vi "Self Configure.vi"(8 "error in":errorcluster, 11 "CrossPoint in":refnum<class "CrossPoint.lvclass">) -> (0 "error out":errorcluster, 3 "CrossPoint out":refnum<class "CrossPoint.lvclass">)   [LabVIEW 2019, in "CrossPoint.lvlib" / "CrossPoint.lvclass"]
doc: "Children of Instruments must override this routine and call the parent method. \nThis routine is implemented to allow each instrument to read its specific configuration keys and implement any default configuration settings.\n\nThis routine already calls Connect and Self Test Routines."
uses:
  Library/CrossPoint.lvclass
  Custom Controls/Configuration Keys.ctl
  Library/CrossPoint.lvclass/CrossPoint.ctl
  builds/Instruments/Instruments.lvlibp/Library/Instruments.lvclass
  builds/Tools/Config.lvlibp/Config.lvclass
  C:/Users/Public/Documents/Development/builds/Tools/Config.lvlibp/Config.lvclass
panel:
  in  "Configuration Keys":T1
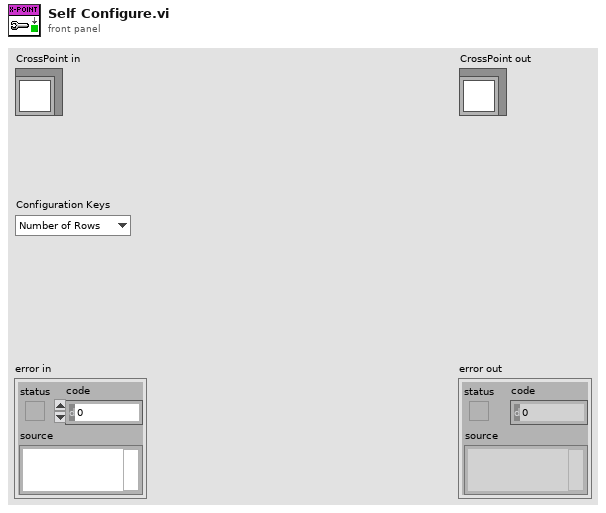
[diagram p1: front panel]
types:
  T1 = typedef "CrossPoint.lvlib/CrossPoint.lvclass/Configuration Keys.ctl" = enum16{"Number of Rows", "Number of Columns"}
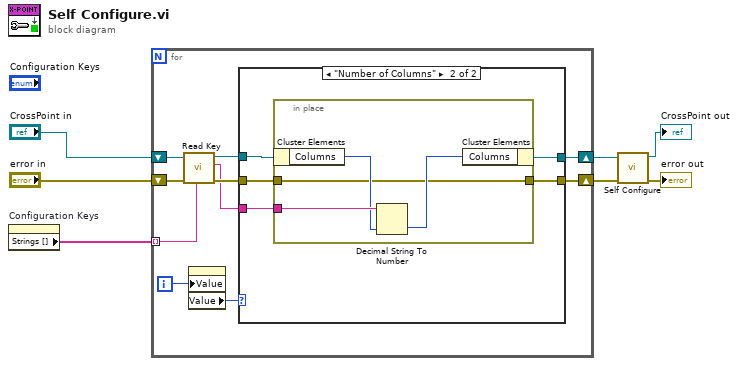
[diagram p0: block diagram]
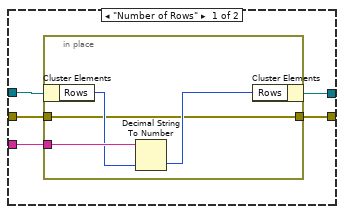
[diagram p2: hidden frame]
diagram:
  n1 = property on="Configuration Keys" class="Enum (strict)"() -> ("Strings []"=w1:string[])  [unwired: 2 in, 2 out]
  n2 = for {
    shift-right: [w10] -> w4
    shift-left: "CrossPoint in" -> [w15]
    shift-right: [w8] -> w2
    shift-left: "error in" -> [w14]
    tunnel: w1 -> [w13] mode=indexing
    i -> [w17]
    n3 = call "Read Key.vi"("Key Name"=w13, "error in"=w14, "Config in"=w15) -> ("error out"=w12:errorcluster, "Key Value"=w9:string, "Config out"=w11:refnum<class "CrossPoint.lvclass">)  [unwired: 6 in]
    n4 = property on="Configuration Keys" class="Enum (strict)"("Value"=w17) -> ("Value"=w16:T1)  [unwired: 2 in, 2 out]
    n5 = case shown="\"Number of Columns\"" w16 {
      tunnel: w12 -> [w20 w29]
      tunnel: w11 -> [w22 w31]
      tunnel: [w21 w30] -> w10
      tunnel: w9 -> [w19 w28]
      tunnel: [w18 w27] -> w8
      frame "Number of Rows" {
        n6 = in-place {
          in-place-border: w20 -> [w23]
          in-place-border: w19 -> [w26]
          in-place-border: [w23] -> w18
          n7 = in-place-cluster #1(w22) -> ("Rows"=w25:u32)
          n8 = Decimal String To Number(string=w26, default (0L)=w25) -> (number=w24:u32)  [unwired: 1 in, 1 out]
          n9 = in-place-cluster #1("Rows"=w24) -> (w21:refnum<class "CrossPoint.lvclass">)
        }
      }
      frame "Number of Columns" {
        n10 = in-place {
          in-place-border: w29 -> [w32]
          in-place-border: w28 -> [w35]
          in-place-border: [w32] -> w27
          n11 = in-place-cluster #2(w31) -> ("Columns"=w34:u32)
          n12 = Decimal String To Number(string=w35, default (0L)=w34) -> (number=w33:u32)  [unwired: 1 in, 1 out]
          n13 = in-place-cluster #2("Columns"=w33) -> (w30:refnum<class "CrossPoint.lvclass">)
        }
      }
    }
  }
  n14 = call-parent "Self Configure.vi"("error in"=w2, "Instruments in"=w4) -> ("error out"=→"error out":errorcluster, "Instruments out"=→"CrossPoint out":refnum<class "CrossPoint.lvclass">)  [unwired: 8 in]
